vi "Single Class_Multiple_State_Self.vi"(0 "State#":i32=1000, 1 "State_Interval_Time(s)":dbl=0.001 min=0.0 max=86400.0 format="%#_13p", 2 "Time Target (s)":dbl=30.0 format="%#_13g", 3 "System_Delay(s)":dbl=0.01 min=0.0 max=86400.0 format="%#_13p") -> ()   [LabVIEW 2021]
uses:
  C:/Program Files (x86)/Hyper State Machine Framework/SSW_Hyper_State_Machine.lvlibp/State_Machine_Class/Main_State_Machine/Hyper_State_Machine.lvclass
  C:/Program Files (x86)/Hyper State Machine Framework/SSW_Hyper_State_Machine.lvlibp/State_Machine_Class/State_Machine_Module.llb/State Machine[].ctl
  C:/Program Files (x86)/Hyper State Machine Framework/SSW_Hyper_State_Machine.lvlibp/State_Machine_Class/State_Machine_Module.llb/Iterval.ctl
  C:/Program Files (x86)/Hyper State Machine Framework/SSW_Hyper_State_Machine.lvlibp/State_Machine_Class/State_Machine_Module.llb/Lock_Unlock.ctl
  C:/Program Files (x86)/Hyper State Machine Framework/SSW_Hyper_State_Machine.lvlibp
panel:
  out "Current State":string
  out "Show_Stop_Button":bool=TRUE
  in  "Unlock":bool
  in  "Reset":bool
  in  "Lock Even":bool
  in  "Lock Odd":bool
  in  "lock All":bool
  in  "Stop":bool
  out "Timing":dbl[](array[numeric])
  out "Lock":bool[](array[boolean])
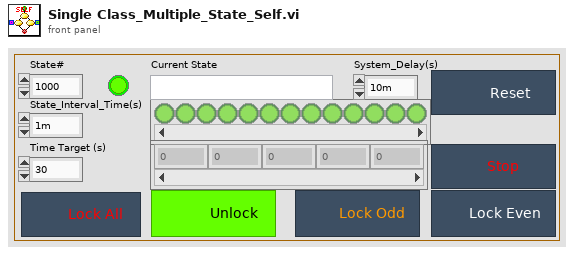
[diagram p1: front panel]
types:
  T1 = typedef "SSW_Hyper_State_Machine.lvlibp/State Machine.ctl" = cluster{"Command":string, "Data":variant}
  T2 = typedef "SSW_Hyper_State_Machine.lvlibp/State Machine[].ctl" = cluster{"Command":string, "Data":variant}[]
  T3 = typedef "SSW_Hyper_State_Machine.lvlibp/Lock_Unlock.ctl" = cluster{"Action_Mode (Get)":enum16{"Set", "Get"}, "Action_Set (False)":bool, "State_In (Wait)":string}
  T4 = typedef "SSW_Hyper_State_Machine.lvlibp/Iterval.ctl" = cluster{"Delay(s)":dbl, "State (Interval_Delay)":string}
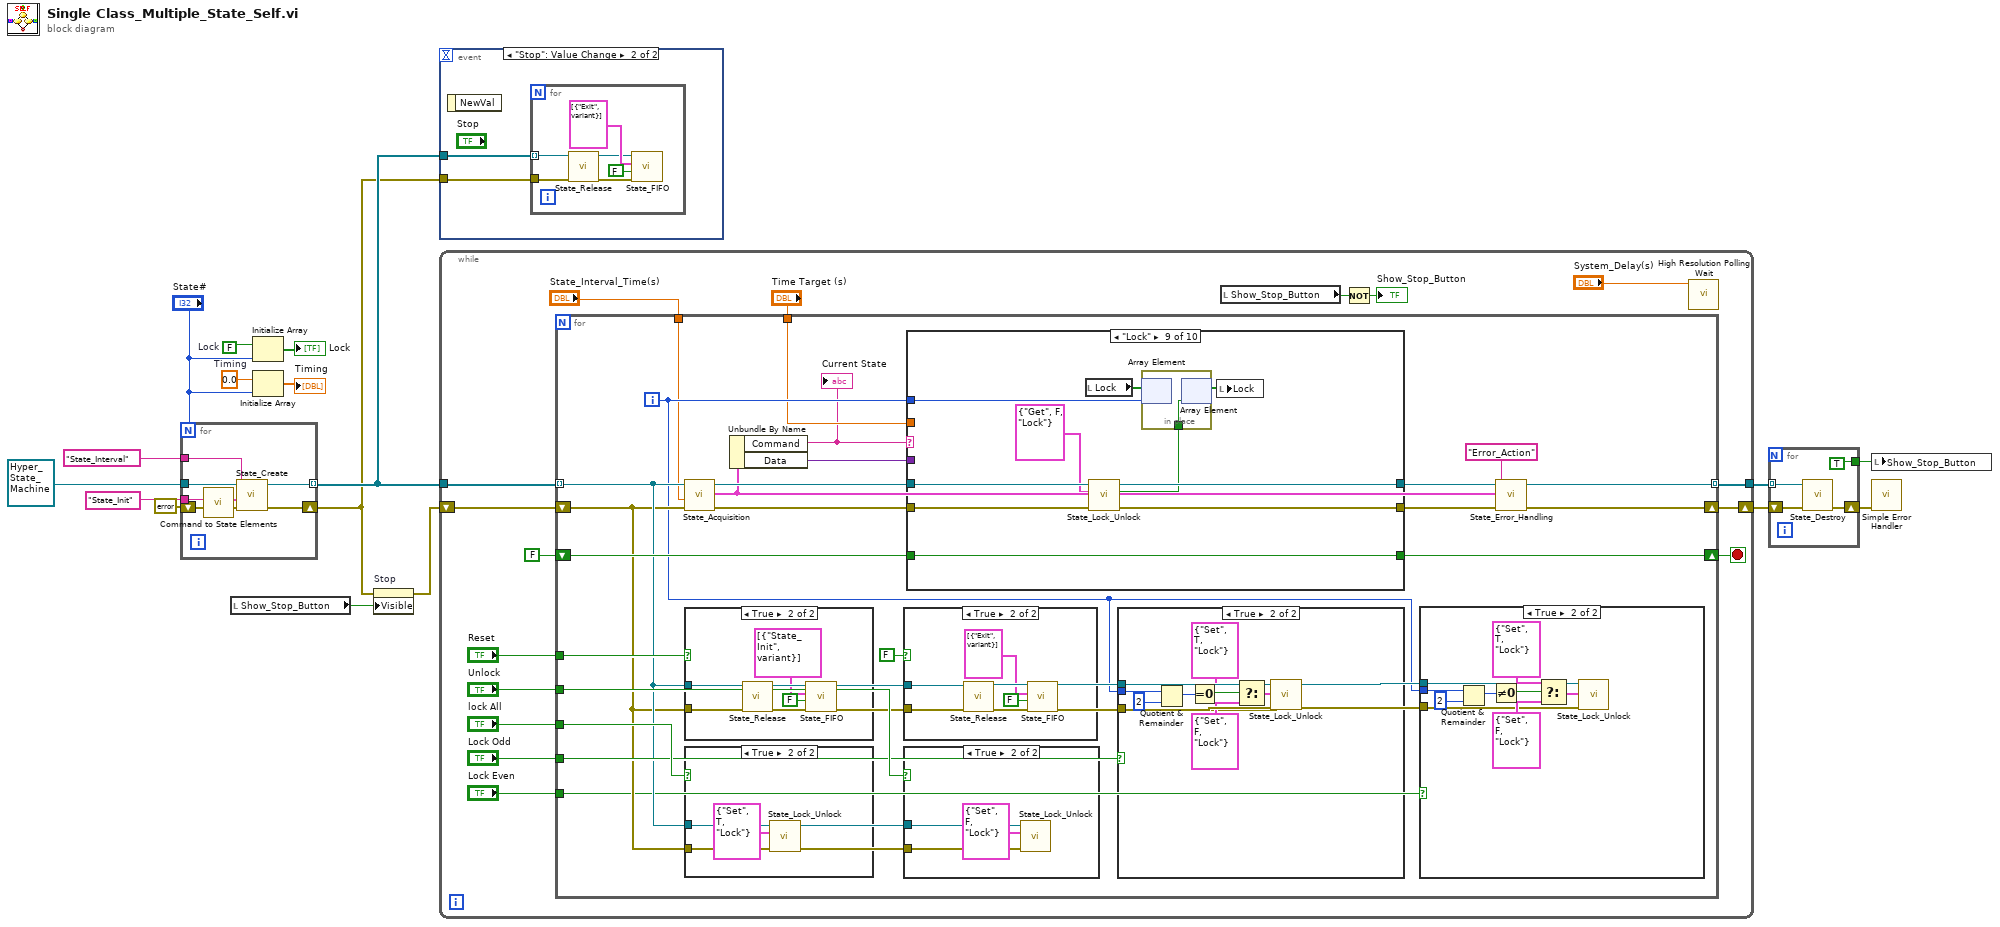
[diagram p0: block diagram]
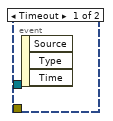
[diagram p2: hidden frame]
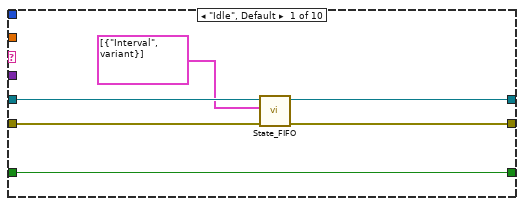
[diagram p9: hidden frame]
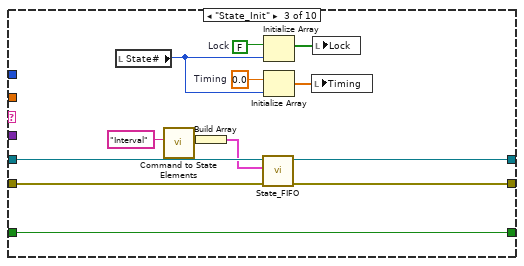
[diagram p11: hidden frame]
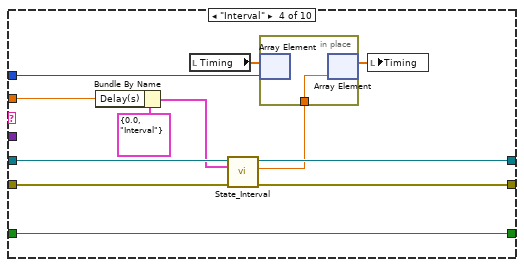
[diagram p12: hidden frame]
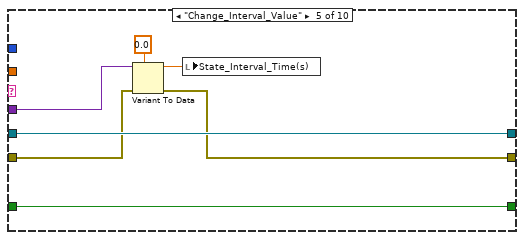
[diagram p13: hidden frame]
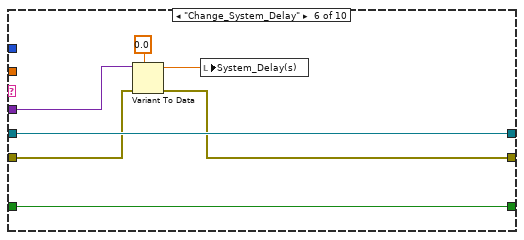
[diagram p14: hidden frame]
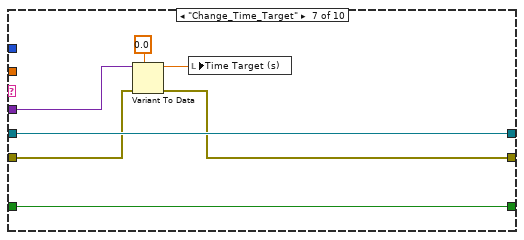
[diagram p15: hidden frame]
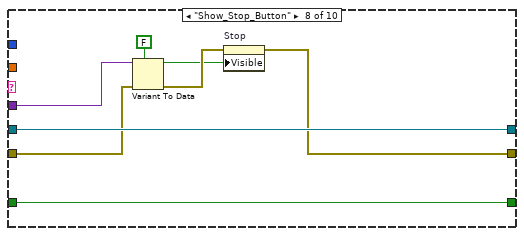
[diagram p16: hidden frame]
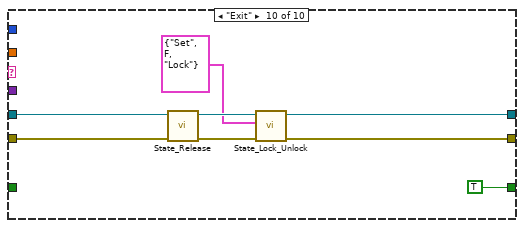
[diagram p17: hidden frame]
diagram:
  w14 = 0.0  # Timing
  w17 = FALSE  # Lock
  n1 = for {
    N: "State#" -> [_]
    tunnel: refnum<class "Hyper_State_Machine.lvclass"> refnum ("SSW_Hyper_State_Machine.lvlibp:Hyper_State_Machine.lvclass") -> [w24]
    tunnel: "State_Init" ("Command") -> [w22]
    tunnel: "State_Interval" ("Core_Interval_Name(State_Interval)") -> [w21]
    shift-right: [w20] -> w5
    shift-left: errorcluster {"status"=FALSE, "code"=0, "source"=""} ("error out") -> [w19]
    tunnel: [w18] -> w6 mode=indexing
    n2 = call "Command to State Elements.vi"("Command"=w22) -> ("Command to State Elements"=w23:T1)  [unwired: 10 in]
    n3 = call-dynamic "State_Create.vi"("error in (no error)"=w19, "Init_State(Option)"=w23, "State_Interval_Name"=w21, "State_Machine_Class in"=w24) -> ("error out"=w20:errorcluster, "State_Machine_Class out"=w18:refnum<class "Hyper_State_Machine.lvclass">)  [unwired: 5 in, 1 out]
  }
  n4 = local read "Show_Stop_Button"() -> (w8:bool)
  n5 = Initialize Array(w17, "State#") -> (→"Lock":bool[])
  n6 = Initialize Array(w14, "State#") -> (→"Timing":dbl[])
  n7 = property on="Stop" class="Bool"(error in=w5, "Visible"=w8) -> (error out=w9:errorcluster)  [unwired: 1 in, 1 out]
  n8 = event shown="[1] \"Stop\": Value Change" {
    selector: _ -> [_ _]
    dyn-events: _ -> [_ _]
    timeout: _ -> [_ _]
    tunnel: w6 -> [_ w26]
    tunnel: w5 -> [_ w25]
    event Timeout {
      n9 = event-data() -> ()  [unwired: 1 in, 3 out]
    }
    event "Stop": Value Change {
      n10 = event-data() -> ()  [unwired: 1 in, 1 out]
      n11 = for {
        tunnel: w26 -> [w28] mode=indexing
        tunnel: w25 -> [w27]
        n12 = call-dynamic "State_Release.vi"("error in (no error)"=w27, "State_Machine_Class in"=w28) -> ("error out"=w30:errorcluster, "State_Machine_Class out"=w29:refnum<class "Hyper_State_Machine.lvclass">)  [unwired: 8 in]
        n13 = call-dynamic "State_FIFO.vi"("error in (no error)"=w30, "State_Interval(Enable)"=FALSE, "State Machine[]"=T2 [{"Command"="Exit", "Data"=variant}], "State_Machine_Class in"=w29) -> ()  [unwired: 6 in, 2 out]
      }
    }
  }
  n14 = while {
    tunnel: w6 -> [w48]
    tunnel: [w44] -> w11
    shift-right: [w43] -> w10
    shift-left: w9 -> [w47]
    stop <- w46 stop-if-true
    n15 = for {
      tunnel: w48 -> [w56] mode=indexing
      shift-right: [w68] -> w43
      shift-left: w47 -> [w55]
      shift-right: [w63] -> w46
      shift-left: FALSE -> [w62]
      tunnel: [w61] -> w44 mode=indexing
      tunnel: "Reset" -> [w60]
      tunnel: "lock All" -> [w59]
      tunnel: "Unlock" -> [w58]
      tunnel: "Lock Odd" -> [w57]
      tunnel: "Lock Even" -> [w54]
      tunnel: "Time Target (s)" -> [w52]
      tunnel: "State_Interval_Time(s)" -> [w51]
      i -> [w53]
      n16 = call-dynamic "State_Acquisition.vi"("error in (no error)"=w55, "State_Interval_Time(s)"=w51, "Main_Machine_State_Class in"=w56) -> ("error out"=w69:errorcluster, "State"=w67:T1, "Main_Machine_State_Class out"=w70:refnum<class "Hyper_State_Machine.lvclass">)  [unwired: 2 in, 4 out]
      n17 = case shown="True" w60 {
        tunnel: w56 -> [_ w107]
        tunnel: w55 -> [_ w103]
        frame False {
        }
        frame True {
          n18 = call-dynamic "State_Release.vi"("error in (no error)"=w103, "State_Machine_Class in"=w107) -> ("error out"=w105:errorcluster, "State_Machine_Class out"=w106:refnum<class "Hyper_State_Machine.lvclass">)  [unwired: 8 in]
          n19 = call-dynamic "State_FIFO.vi"("error in (no error)"=w105, "State_Interval(Enable)"=FALSE, "State Machine[]"=T2 [{"Command"="State_Init", "Data"=variant}], "State_Machine_Class in"=w106) -> ()  [unwired: 6 in, 2 out]
        }
      }
      n20 = case shown="True" w59 {
        tunnel: w56 -> [_ w95]
        tunnel: w55 -> [_ w94]
        frame False {
        }
        frame True {
          n21 = call-dynamic "State_Lock_Unlock.vi"("error in (no error)"=w94, "Parameter"=T3 {"Action_Mode (Get)"=enum."Set", "Action_Set (False)"=TRUE, "State_In (Wait)"="Lock"}, "State_Machine_Class in"=w95) -> ()  [unwired: 6 in, 3 out]
        }
      }
      n22 = Unbundle By Name(w67) -> ("Command"=w49:string, "Data"=w71:variant)
      "Current State" <- w49
      n23 = case shown="True" FALSE {
        tunnel: w56 -> [_ w101]
        tunnel: w55 -> [_ w97]
        frame False {
        }
        frame True {
          n24 = call-dynamic "State_Release.vi"("error in (no error)"=w97, "State_Machine_Class in"=w101) -> ("error out"=w99:errorcluster, "State_Machine_Class out"=w100:refnum<class "Hyper_State_Machine.lvclass">)  [unwired: 8 in]
          n25 = call-dynamic "State_FIFO.vi"("error in (no error)"=w99, "State_Interval(Enable)"=FALSE, "State Machine[]"=T2 [{"Command"="Exit", "Data"=variant}], "State_Machine_Class in"=w100) -> ()  [unwired: 6 in, 2 out]
        }
      }
      n26 = case shown="True" w58 {
        tunnel: w56 -> [_ w91]
        tunnel: w55 -> [_ w92]
        frame False {
        }
        frame True {
          n27 = call-dynamic "State_Lock_Unlock.vi"("error in (no error)"=w92, "Parameter"=T3 {"Action_Mode (Get)"=enum."Set", "Action_Set (False)"=FALSE, "State_In (Wait)"="Lock"}, "State_Machine_Class in"=w91) -> ()  [unwired: 6 in, 3 out]
        }
      }
      n28 = case shown="\"Lock\"" w49 {
        tunnel: w71 -> [_ _ _ _ w148 w155 w162 w170 _ _]
        tunnel: w70 -> [w112 w116 w128 w135 w149 w156 w163 w171 w181 w189]
        tunnel: w69 -> [w111 w115 w126 w134 w147 w154 w161 w169 w180 w188]
        tunnel: [w110 w116 w127 w132 w149 w156 w163 w171 w179 w185] -> w65
        tunnel: [w109 w115 w125 w131 w146 w153 w160 w164 w178 w184] -> w64
        tunnel: w53 -> [_ _ _ w141 _ _ _ _ w174 _]
        tunnel: [w113 w114 w129 w138 w144 w151 w158 w168 w176 TRUE] -> w63
        tunnel: w62 -> [w113 w114 w129 w138 w144 w151 w158 w168 w176 _]
        tunnel: w52 -> [_ _ _ w137 _ _ _ _ _ _]
        frame "Idle", Default {
          n29 = call-dynamic "State_FIFO.vi"("error in (no error)"=w111, "State Machine[]"=T2 [{"Command"="Interval", "Data"=variant}], "State_Machine_Class in"=w112) -> ("error out"=w109:errorcluster, "State_Machine_Class out"=w110:refnum<class "Hyper_State_Machine.lvclass">)  [unwired: 7 in]
        }
        frame "State_Interval" {
          # "Execute Every Define of State Interval Time"
        }
        frame "State_Init" {
          w121 = 0.0  # Timing
          w120 = FALSE  # Lock
          n30 = local read "State#"() -> (w119:i32)
          n31 = call "Command to State Elements.vi"("Command"="Interval") -> ("Command to State Elements"=w123:T1)  [unwired: 10 in]
          n32 = Build Array(w123) -> (w122:T1[])
          n33 = call-dynamic "State_FIFO.vi"("error in (no error)"=w126, "State Machine[]"=w122, "State_Machine_Class in"=w128) -> ("error out"=w125:errorcluster, "State_Machine_Class out"=w127:refnum<class "Hyper_State_Machine.lvclass">)  [unwired: 7 in]
          n34 = Initialize Array(w120, w119) -> (w117:bool[])
          n35 = Initialize Array(w121, w119) -> (w118:dbl[])
          n36 = local write "Timing"(w118) -> ()
          n37 = local write "Lock"(w117) -> ()
        }
        frame "Interval" {
          n38 = Bundle By Name(cluster=T4 {"Delay(s)"=0.0, "State (Interval_Delay)"="Interval"} ("Parameter"), "Delay(s)"=w137) -> (w133:T4)
          n39 = local read "Timing"() -> (w140:dbl[])
          n40 = call-dynamic "State_Interval.vi"("error in (no error)"=w134, "Parameter"=w133, "State_Machine_Class in"=w135) -> ("error out"=w131:errorcluster, "Elapsed Time(s)"=w130:dbl, "State_Machine_Class out"=w132:refnum<class "Hyper_State_Machine.lvclass">)  [unwired: 6 in]
          n41 = in-place {
            in-place-border: w130 -> [w142]
            n42 = in-place-array #1(w140, w141) -> ()  [unwired: 1 out]
            n43 = in-place-array #1(w142) -> (w139:dbl[])  [unwired: 1 out]
          }
          n44 = local write "Timing"(w139) -> ()
        }
        frame "Change_Interval_Value" {
          n45 = Variant To Data(error in=w147, type=0.0 ("Time Target (s)"), Variant=w148) -> (data=w143:dbl, error out=w146:errorcluster)
          n46 = local write "State_Interval_Time(s)"(w143) -> ()
        }
        frame "Change_System_Delay" {
          n47 = Variant To Data(error in=w154, type=0.0 ("Time Target (s)"), Variant=w155) -> (data=w150:dbl, error out=w153:errorcluster)
          n48 = local write "System_Delay(s)"(w150) -> ()
        }
        frame "Change_Time_Target" {
          n49 = Variant To Data(error in=w161, type=0.0 ("Time Target (s)"), Variant=w162) -> (data=w157:dbl, error out=w160:errorcluster)
          n50 = local write "Time Target (s)"(w157) -> ()
        }
        frame "Show_Stop_Button" {
          n51 = Variant To Data(error in=w169, type=FALSE, Variant=w170) -> (data=w165:bool, error out=w166:errorcluster)
          n52 = property on="Stop" class="Bool"(error in=w166, "Visible"=w165) -> (error out=w164:errorcluster)  [unwired: 1 in, 1 out]
        }
        frame "Lock" {
          n53 = local read "Lock"() -> (w172:bool[])
          n54 = call-dynamic "State_Lock_Unlock.vi"("error in (no error)"=w180, "Parameter"=T3 {"Action_Mode (Get)"=enum."Get", "Action_Set (False)"=FALSE, "State_In (Wait)"="Lock"}, "State_Machine_Class in"=w181) -> ("error out"=w178:errorcluster, "Action_Get"=w173:bool, "State_Machine_Class out"=w179:refnum<class "Hyper_State_Machine.lvclass">)  [unwired: 6 in]
          n55 = in-place {
            in-place-border: w173 -> [w182]
            n56 = in-place-array #2(w172, w174) -> ()  [unwired: 1 out]
            n57 = in-place-array #2(w182) -> (w175:bool[])  [unwired: 1 out]
          }
          n58 = local write "Lock"(w175) -> ()
        }
        frame "Exit" {
          n59 = call-dynamic "State_Release.vi"("error in (no error)"=w188, "State_Machine_Class in"=w189) -> ("error out"=w186:errorcluster, "State_Machine_Class out"=w187:refnum<class "Hyper_State_Machine.lvclass">)  [unwired: 8 in]
          n60 = call-dynamic "State_Lock_Unlock.vi"("error in (no error)"=w186, "Parameter"=T3 {"Action_Mode (Get)"=enum."Set", "Action_Set (False)"=FALSE, "State_In (Wait)"="Lock"}, "State_Machine_Class in"=w187) -> ("error out"=w184:errorcluster, "State_Machine_Class out"=w185:refnum<class "Hyper_State_Machine.lvclass">)  [unwired: 6 in, 1 out]
        }
      }
      n61 = case shown="True" w57 {
        tunnel: w53 -> [_ w83]
        tunnel: w56 -> [_ w82]
        tunnel: w55 -> [_ w81]
        frame False {
        }
        frame True {
          n62 = Quotient & Remainder(x=w83, y=2) -> (x-y*floor(x/y)=w88:i32)  [unwired: 1 out]
          n63 = Equal To 0?(x=w88) -> (x = 0?=w87:bool)
          n64 = Select(t=T3 {"Action_Mode (Get)"=enum."Set", "Action_Set (False)"=TRUE, "State_In (Wait)"="Lock"} ("Parameter"), s=w87, f=T3 {"Action_Mode (Get)"=enum."Set", "Action_Set (False)"=FALSE, "State_In (Wait)"="Lock"} ("Parameter")) -> (s? t:f=w84:T3)
          n65 = call-dynamic "State_Lock_Unlock.vi"("error in (no error)"=w81, "Parameter"=w84, "State_Machine_Class in"=w82) -> ()  [unwired: 6 in, 3 out]
        }
      }
      n66 = case shown="True" w54 {
        tunnel: w53 -> [_ w74]
        tunnel: w56 -> [_ w73]
        tunnel: w55 -> [_ w72]
        frame False {
        }
        frame True {
          n67 = Quotient & Remainder(x=w74, y=2) -> (x-y*floor(x/y)=w79:i32)  [unwired: 1 out]
          n68 = Not Equal To 0?(x=w79) -> (x != 0?=w78:bool)
          n69 = Select(t=T3 {"Action_Mode (Get)"=enum."Set", "Action_Set (False)"=TRUE, "State_In (Wait)"="Lock"} ("Parameter"), s=w78, f=T3 {"Action_Mode (Get)"=enum."Set", "Action_Set (False)"=FALSE, "State_In (Wait)"="Lock"} ("Parameter")) -> (s? t:f=w75:T3)
          n70 = call-dynamic "State_Lock_Unlock.vi"("error in (no error)"=w72, "Parameter"=w75, "State_Machine_Class in"=w73) -> ()  [unwired: 6 in, 3 out]
        }
      }
      n71 = call-dynamic "State_Error_Handling.vi"("error in (no error)"=w64, "Reply_State_Name"="Error_Action", "Handling_State(State_Acquisition)"=w67, "State_Machine_Class in"=w65) -> ("error out"=w68:errorcluster, "State_Machine_Class out"=w61:refnum<class "Hyper_State_Machine.lvclass">)  [unwired: 6 in]
    }
    n72 = local read "Show_Stop_Button"() -> (w34:bool)
    n73 = Not(x=w34) -> (.not. x?=→"Show_Stop_Button":bool)
    n74 = call <vilib>:"High Resolution Polling Wait.vi"("seconds to wait"="System_Delay(s)") -> ()  [unwired: 10 in, 1 out]
  }
  n75 = for {
    shift-right: [w194] -> w12
    shift-left: w10 -> [w193]
    tunnel: w11 -> [w192] mode=indexing
    tunnel: [TRUE ("Show_Stop_Button")] -> w7
    n76 = call-dynamic "State_Destroy.vi"("error in (no error)"=w193, "State_Machine_Class in"=w192) -> ("error out"=w194:errorcluster)  [unwired: 9 in]
  }
  n77 = local write "Show_Stop_Button"(w7) -> ()
  n78 = call <vilib>:"Simple Error Handler.vi"("error in (no error)"=w12) -> ()  [unwired: 4 in, 5 out]
